vi "DCA Determine Channel Type From Name.vi"(10 "Channel Name":string) -> (2 "Channel Type":T1)   [LabVIEW 2011]
uses:
  TypeDefs/DCA Channel Type.ctl
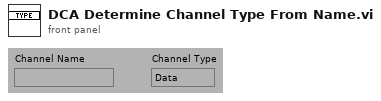
[diagram p1: front panel]
types:
  T1 = typedef "DCA Channel Type.ctl" = enum16{"Data", "Limit", "Invalid", "Topology"}
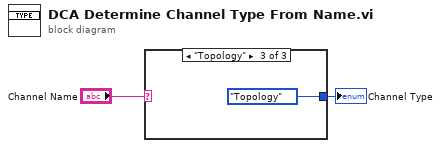
[diagram p0: block diagram]
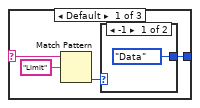
[diagram p2: hidden frame]
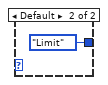
[diagram p3: hidden frame]
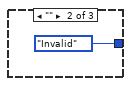
[diagram p4: hidden frame]
diagram:
  n1 = case shown="\"Topology\"" "Channel Name" {
    selector: "Channel Name" -> [w3 _ _]
    tunnel: [w4 DCA_Channel_Type."Invalid" ("Channel Type") DCA_Channel_Type."Topology" ("Channel Type")] -> w2
    frame Default {
      n2 = Match Pattern(string=w3, regular expression="Limit") -> (offset past match=w5:i32)  [unwired: 4 out]
      n3 = case shown="-1" w5 {
        tunnel: [DCA_Channel_Type."Data" ("Channel Type") DCA_Channel_Type."Limit" ("Channel Type")] -> w4
        frame -1 {
        }
        frame Default {
        }
      }
    }
    frame "" {
    }
    frame "Topology" {
    }
  }
  "Channel Type" <- w2
